vi "IT8800-Query Input.vi"(8 "error in":errorcluster, 11 "IT8800 Setting In In":T1={"VISA Resource Name"="", "Baud Rate"=19200, "Stop Bits"=20, "Wait For Read(ms)"=0} {"Stop Bits" items=["1.0"=10, "2.0"=20]; "Baud Rate" items=["2400"=2400, "4800"=4800, "9600"=9600, "19200"=19200]}) -> (0 "error out":errorcluster, 2 "Input?":bool, 3 "IT8800 Setting In Out":T1={"VISA Resource Name"="", "Baud Rate"=19200, "Stop Bits"=20, "Wait For Read(ms)"=0} {"Stop Bits" items=["1.0"=10, "2.0"=20]; "Baud Rate" items=["2400"=2400, "4800"=4800, "9600"=9600, "19200"=19200]})   [LabVIEW 2018]
uses:
  Data Def/IT8800-Setting.ctl
panel:
  out "Response":string
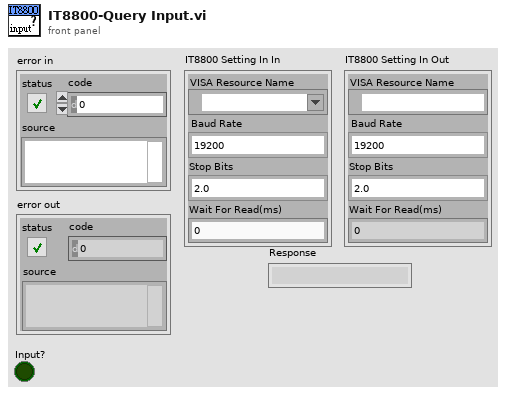
[diagram p1: front panel]
types:
  T1 = typedef "IT8800-Setting.ctl" = cluster{"VISA Resource Name":refnum<visa-resource-name>, "Baud Rate":u32, "Stop Bits":u16, "Wait For Read(ms)":u32}
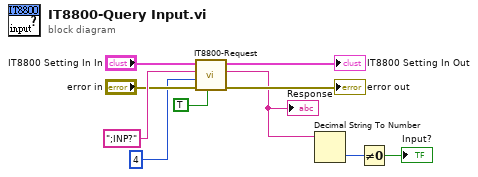
[diagram p0: block diagram]
diagram:
  n1 = call "IT8800-Request.vi"("Response?"=TRUE, "error in"="error in", "byte count"=u32 4, "Command"=";INP?", "IT8800 Setting In In"="IT8800 Setting In In") -> ("error out"=→"error out":errorcluster, "Response"=w5:string, "IT8800 Setting In Out"=→"IT8800 Setting In Out":T1)  [unwired: 4 in]
  "Response" <- w5
  n2 = Decimal String To Number(string=w5) -> (number=w4:i32)  [unwired: 2 in, 1 out]
  n3 = Not Equal To 0?(x=w4) -> (x != 0?=→"Input?":bool)
